vi "initialise.vi"(8 "error in (no error)":errorcluster, 9 "error boolean":refnum<vi>, 10 "error file store path":path, 11 "ErrorController in":refnum<class "ErrorController.lvclass">) -> (0 "error out":errorcluster, 3 "ErrorController out":refnum<class "ErrorController.lvclass">)   [LabVIEW 2010, in "ErrorController.lvclass"]
doc: "The dynamic dispatch-version of this VI initalises the plug-in object by allocating and initalising any dynamic resources need."
uses:
  ErrorController.lvclass
  error_cluster.ctl
  queue controller.ctl
  ErrorController.lvclass/ErrorController.ctl
  class_data.vi
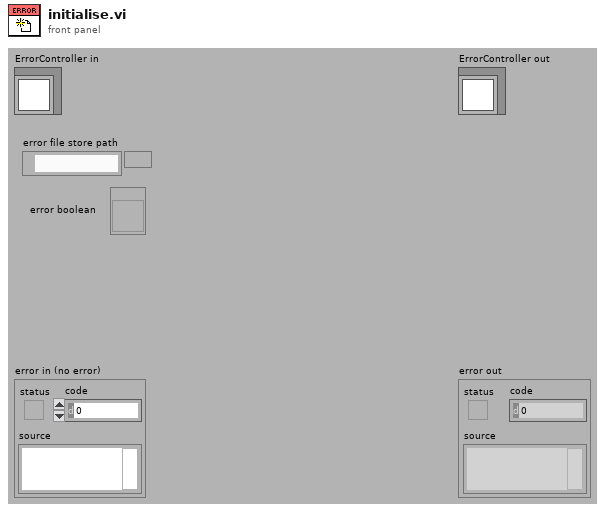
[diagram p1: front panel]
types:
  T1 = enum16{"open", "replace", "create", "open or create", "replace or create", "replace or create with confirmation"}
  T2 = typedef "ErrorController.lvclass/error_cluster.ctl" = cluster{"error out":errorcluster, "call chain":string[], "additional message":string, "terminate?":bool, "concatenated string":string}
  T3 = typedef "ErrorController.lvclass/queue controller.ctl" = refnum<queue>
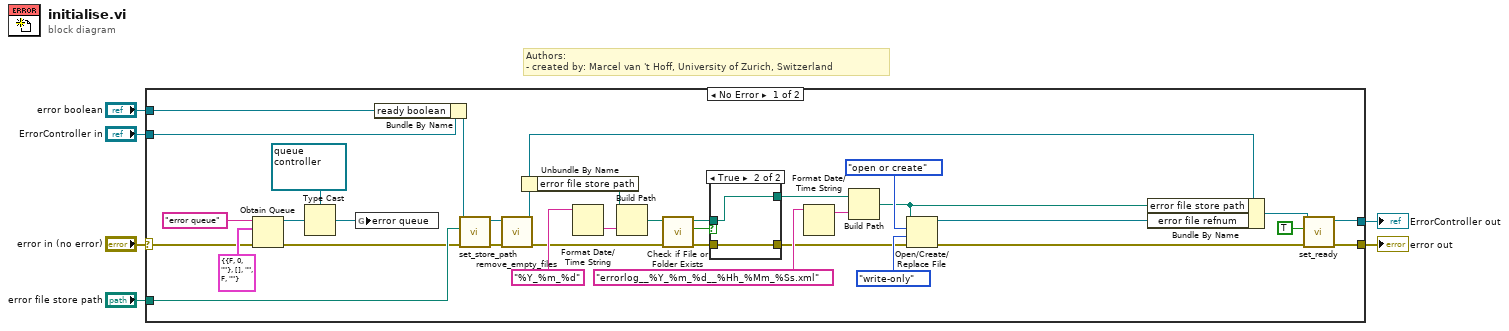
[diagram p0: block diagram]
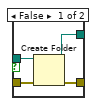
[diagram p2: hidden frame]
diagram:
  # "Authors: \n- created by: Marcel van 't Hoff, University of Zurich, Switzerland"
  n1 = case shown="No Error" "error in (no error)" {
    selector: "error in (no error)" -> [w14 w49]
    tunnel: [w7 w49] -> w6
    tunnel: [w8 w48] -> w5
    tunnel: "ErrorController in" -> [w18 w48]
    tunnel: "error file store path" -> [w15 _]
    tunnel: "error boolean" -> [w16 _]
    frame No Error {
      n2 = Obtain Queue(name (unnamed)="error queue", element data type=T2 {"error out"={"status"=FALSE, "code"=0, "source"=""}, "call chain"=[], "additional message"="", "terminate?"=FALSE, "concatenated string"=""} ("error cluster"), error in (no error)=w14) -> (queue out=w39:refnum<queue>, error out=w13:errorcluster)  [unwired: 2 in, 1 out]
      n3 = Type Cast(type=T3 refnum ("error queue"), x=w39) -> (*(type *) &x=w37:T3)
      n4 = global write "class_data.vi" "error queue"(w37) -> ()
      n5 = Bundle By Name(cluster=w18, "ready boolean"=w16) -> (w17:refnum<class "ErrorController.lvclass">)
      n6 = call-dynamic "set_store_path.vi"("error in (no error)"=w13, "error file store path"=w15, "ErrorController in"=w17) -> ("error out"=w20:errorcluster, "ErrorController out"=w21:refnum<class "ErrorController.lvclass">)  [unwired: 7 in]
      n7 = call-dynamic "remove_empty_files.vi"("error in (no error)"=w20, "ErrorController in"=w21) -> ("error out"=w12:errorcluster, "ErrorController out"=w19:refnum<class "ErrorController.lvclass">)  [unwired: 8 in]
      n8 = Unbundle By Name(w19) -> ("error file store path"=w33:path)
      n9 = Format Date/Time String(time format string (%c)="%Y_%m_%d") -> (date/time string=w34:string)  [unwired: 2 in]
      n10 = Build Path(base path=w33, name or relative path=w34) -> (appended path=w27:path)
      n11 = call <vilib>:"Check if File or Folder Exists.vi"("error in (no error)"=w12, "path"=w27) -> ("error out"=w25:errorcluster, "file or folder exists?"=w24:bool, "dup path"=w26:path)  [unwired: 7 in]
      n12 = case shown="True" w24 {
        tunnel: [w45 w46] -> w29
        tunnel: [w44 w47] -> w28
        tunnel: w26 -> [w43 w46]
        tunnel: w25 -> [w42 w47]
        frame False {
          n13 = Create Folder(path (use dialog)=w43, error in=w42) -> (created path=w45:path, error out=w44:errorcluster)  [unwired: 1 in, 1 out]
        }
        frame True {
        }
      }
      n14 = Format Date/Time String(time format string (%c)="errorlog__%Y_%m_%d__%Hh_%Mm_%Ss.xml") -> (date/time string=w30:string)  [unwired: 2 in]
      n15 = Build Path(base path=w29, name or relative path=w30) -> (appended path=w23:path)
      n16 = Open/Create/Replace File(file path (use dialog)=w23, error in=w28, operation (0:open)=T1."open or create", access (0:read/write)=enum16{"read/write", "read-only", "write-only"}."write-only") -> (refnum out=w22:refnum<file>, error out=w9:errorcluster)  [unwired: 2 in, 1 out]
      n17 = Bundle By Name(cluster=w19, "error file store path"=w23, "error file refnum"=w22) -> (w10:refnum<class "ErrorController.lvclass">)
      n18 = call-dynamic "set_ready.vi"("error in (no error)"=w9, "ready?"=TRUE, "ErrorController in"=w10) -> ("error out"=w7:errorcluster, "ErrorController out"=w8:refnum<class "ErrorController.lvclass">)  [unwired: 7 in]
    }
    frame Error {
    }
  }
  "error out" <- w6
  "ErrorController out" <- w5
